vi "SVT Get Octave Subset (1 Ch).vi"(0 "octave spectrum":T5 {"band power" format="%.2f"; "nominal frequencies [Hz]" format="%.2f"}, 5 "frequency range [Hz]":cluster{"start":dbl, "stop":dbl}={"start"=-1.0, "stop"=-1.0} {"stop" format="%.2f"; "start" format="%.2f"}, 9 "octave info in":T1={"standard"=enum."ANSI S1.11", "bandwidth"=enum."1 octave", "low band"=0, "high band"=0, "weighting filter"=0, "dB reference"=0.0, "dB On"=FALSE, "unit label"="", "channel name"="", "description"="", "engineering units"=1, "custom label"="", "spectrum type"=enum."magnitude", "spectral density"=FALSE, "filters settled"=FALSE} {"engineering units" items=["custom..."=0, "V"=1, "A"=21, "C"=30, "pC"=31, "s"=32, "-"=29, "Pa"=2, "N"=20, "g"=3, "m/s^2"=4, "m/s"=5, "m"=6, "mm/s"=12, "mm"=13, "micron/s"=14, "micron"=15, "in/s^2"=7, "in/s"=8, "in"=9, "mil/s"=10, "mil"=11, "rad/s^2"=16, "rad/s"=17, "rad"=18, "deg/s^2"=26, "deg/s"=27, "deg"=28, "RPM"=22, "cycle/s^2"=23, "Hz"=24, "cycle"=25, "strain"=19]; "dB reference" format="%.2e"; "weighting filter" items=["Linear", "A-weighting", "B-weighting", "C-weighting", "ITU-R 468-4", "Dolby", "CCITT", "C-message", "Wb", "Wc", "Wd", "We", "Wf", "Wh", "Wj", "Wk", "Wm", "AES17 20 kHz lowpass", "AES17 40 kHz lowpass", "AES17 20 kHz highpass", "AES17 40 kHz highpass"]}, 11 "error in (no error)":errorcluster) -> (4 "octave spectrum subset":T5 {"band power" format="%.2f"; "nominal frequencies [Hz]" format="%.2f"}, 6 "unit label":string, 8 "total band power":dbl=nan, 10 "octave info out":T1={"standard"=enum."ANSI S1.11", "bandwidth"=enum."1 octave", "low band"=0, "high band"=0, "weighting filter"=0, "dB reference"=0.0, "dB On"=FALSE, "unit label"="", "channel name"="", "description"="", "engineering units"=1, "custom label"="", "spectrum type"=enum."magnitude", "spectral density"=FALSE, "filters settled"=FALSE} {"engineering units" items=["custom..."=0, "V"=1, "A"=21, "C"=30, "pC"=31, "s"=32, "-"=29, "Pa"=2, "N"=20, "g"=3, "m/s^2"=4, "m/s"=5, "m"=6, "mm/s"=12, "mm"=13, "micron/s"=14, "micron"=15, "in/s^2"=7, "in/s"=8, "in"=9, "mil/s"=10, "mil"=11, "rad/s^2"=16, "rad/s"=17, "rad"=18, "deg/s^2"=26, "deg/s"=27, "deg"=28, "RPM"=22, "cycle/s^2"=23, "Hz"=24, "cycle"=25, "strain"=19]; "dB reference" format="%.2e"; "weighting filter" items=["Linear", "A-weighting", "B-weighting", "C-weighting", "ITU-R 468-4", "Dolby", "CCITT", "C-message", "Wb", "Wc", "Wd", "We", "Wf", "Wh", "Wj", "Wk", "Wm", "AES17 20 kHz lowpass", "AES17 40 kHz lowpass", "AES17 20 kHz highpass", "AES17 40 kHz highpass"]}, 15 "error out":errorcluster)   [LabVIEW 2017, in "SoundVib_Octave_2014 standard.lvlib"]
doc: "Extracts the subset of the <B>octave spectrum</B> specified by <B>frequency range</B> for a single channel or N channels. Wire data to the <B>octave spectrum</B> input to determine the polymorphic instance to use or manually select the instance."
uses:
  <vilib>/addons/Sound and Vibration/svt_Octave/SoundVib_Octave_2014 standard.lvlib
  <vilib>/addons/_NISVFA/_Shared subVIs/Controls/svc_Octave Info.ctl
  <vilib>/addons/_NISVFA/_Shared subVIs/Controls/svc_Octave Standard.ctl
  <vilib>/addons/_NISVFA/_Shared subVIs/Controls/svc_Weighting Filter Text Ring.ctl
  <vilib>/addons/_NISVFA/_Shared subVIs/Controls/svc_Engineering Units Text Ring.ctl
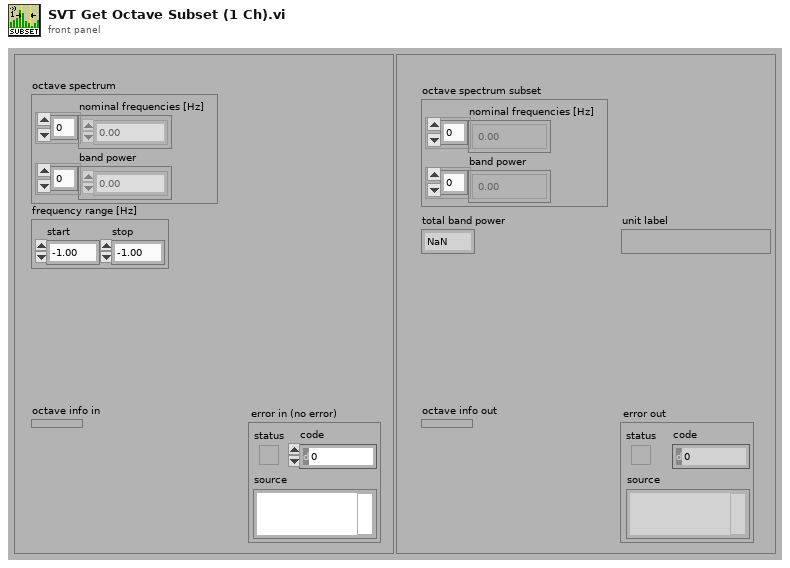
[diagram p1: front panel]
types:
  T1 = typedef "svc_Octave Info.ctl" = cluster{"standard":T2, "bandwidth":enum16{"1 octave", "1/3 octave", "1/6 octave", "1/12 octave", "1/24 octave"}, "low band":i32, "high band":i32, "weighting filter":T3, "dB reference":dbl, "dB On":bool, "unit label":string, "channel name":string, "description":string, "engineering units":T4, "custom label":string, "spectrum type":enum16{"power", "magnitude"}, "spectral density":bool, "filters settled":bool}
  T2 = typedef "svc_Octave Standard.ctl" = enum16{"ANSI S1.11", "IEC 61260"}
  T3 = typedef "svc_Weighting Filter Text Ring.ctl" = u16
  T4 = typedef "svc_Engineering Units Text Ring.ctl" = u16
  T5 = cluster{"nominal frequencies [Hz]":dbl[], "band power":dbl[]}
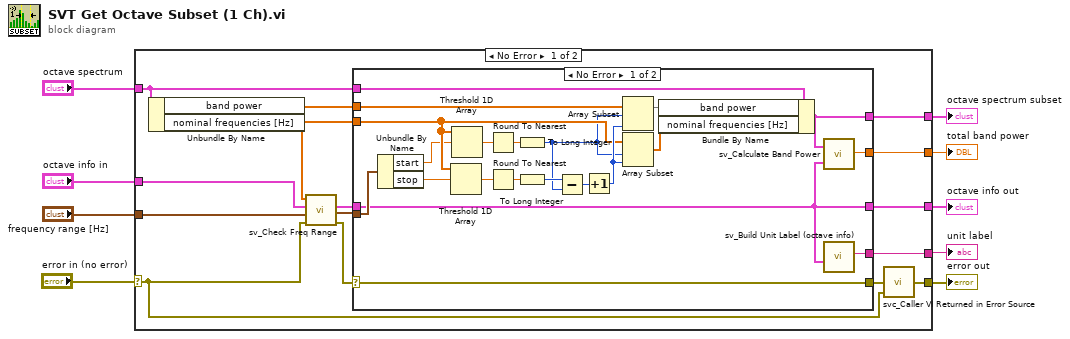
[diagram p0: block diagram]
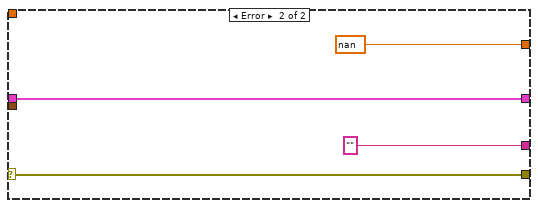
[diagram p2: hidden frame]
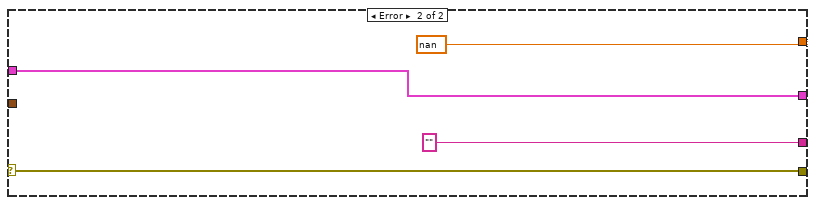
[diagram p3: hidden frame]
diagram:
  n1 = case shown="No Error" "error in (no error)" {
    selector: "error in (no error)" -> [w10 w53]
    tunnel: "frequency range [Hz]" -> [w23 _]
    tunnel: "octave spectrum" -> [w24 _]
    tunnel: "octave info in" -> [w15 w50]
    tunnel: [w11 w53] -> w9
    tunnel: [w18 "" ("frequency range string")] -> w4
    tunnel: [w20 w50] -> w3
    tunnel: [w19 _] -> w2
    tunnel: [w17 nan ("start frequency")] -> w1
    frame No Error {
      n2 = Unbundle By Name(w24) -> ("band power"=w22:dbl[], "nominal frequencies [Hz]"=w21:dbl[])
      n3 = call <vilib>:"sv_Check Freq Range.vi"("error in (no error)"=w10, "range in"=w23, "octave info in"=w15, "nominal frequencies [Hz]"=w21) -> ("error out"=w14:errorcluster, "range out"=w16:cluster{"start":dbl, "stop":dbl}, "octave info out"=w13:T1)  [unwired: 4 in, 1 out]
      n4 = case shown="No Error" w14 {
        selector: w14 -> [w34 w47]
        tunnel: w24 -> [w45 _]
        tunnel: w22 -> [w44 _]
        tunnel: w21 -> [w31 _]
        tunnel: w16 -> [w39 _]
        tunnel: [w33 w46] -> w20
        tunnel: [w40 _] -> w19
        tunnel: [w34 w47] -> w12
        tunnel: [w32 "" ("unit label")] -> w18
        tunnel: [w41 nan ("total band power [dB EU]")] -> w17
        tunnel: w13 -> [w33 w46]
        frame No Error {
          n5 = Unbundle By Name(w39) -> ("start"=w30:dbl, "stop"=w38:dbl)
          n6 = Threshold 1D Array(2:w38, 3:w31) -> (0:w37:dbl)  [unwired: 1 in]
          n7 = Threshold 1D Array(2:w30, 3:w31) -> (0:w29:dbl)  [unwired: 1 in]
          n8 = Round To Nearest(number=w29) -> (nearest integer value=w26:dbl)
          n9 = Round To Nearest(number=w37) -> (nearest integer value=w25:dbl)
          n10 = To Long Integer(number=w26) -> (32bit integer=w27:i32)
          n11 = To Long Integer(number=w25) -> (32bit integer=w28:i32)
          n12 = Subtract(x=w28, y=w27) -> (x-y=w36:i32)
          n13 = Increment(x=w36) -> (x+1=w35:i32)
          n14 = Array Subset(array=w44, index=w27, length=w35) -> (w43:dbl[])
          n15 = Array Subset(array=w31, index=w27, length=w35) -> (w42:dbl[])
          n16 = Bundle By Name(cluster=w45, "band power"=w43, "nominal frequencies [Hz]"=w42) -> (w40:T5)
          n17 = call <vilib>:"sv_Calculate Band Power.vi"("octave info"=w33, "octave spectrum"=w40) -> ("total band power"=w41:dbl)
          n18 = call <vilib>:"sv_Build Unit Label (octave info).vi"("octave info"=w33) -> ("unit label"=w32:string)  [unwired: 8 in, 2 out]
        }
        frame Error {
        }
      }
      n19 = call <vilib>:"svc_Caller VI Returned in Error Source.vi"("warning input to caller"=w10, "error in (no error)"=w12) -> ("error out"=w11:errorcluster)  [unwired: 3 in]
    }
    frame Error {
    }
  }
  "error out" <- w9
  "octave spectrum subset" <- w2
  "octave info out" <- w3
  "unit label" <- w4
  "total band power" <- w1
